vi "Configure List State.vi"(8 "error in":errorcluster, 10 "State":u16(ring) items=["OFF", " LIST1", " LIST2", " LIST3", " LIST4", " LIST5"], 11 "VISA resource name":refnum<visa-resource-name>) -> (0 "error out":errorcluster, 3 "VISA resource name out":refnum<visa-resource-name>)   [LabVIEW 2015, in "IT-M7700.lvlib"]
doc: "This command is used to set the mode of the List.\n<b>State</b>\n1~5 means to open the List function and call list1-list5, and OFF means to close the List function."
uses:
  <instrlib>/IT-M7700/IT-M7700.lvlib
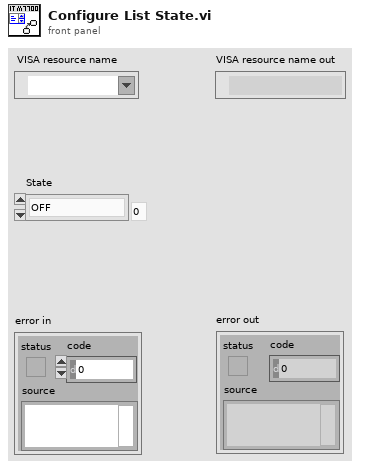
[diagram p1: front panel]
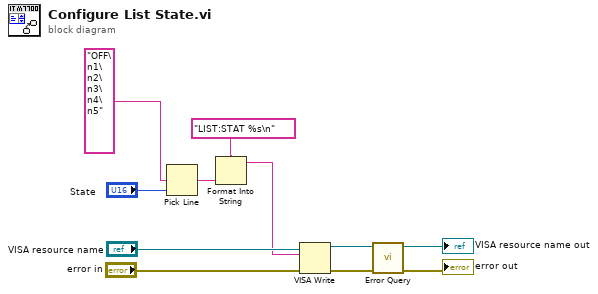
[diagram p0: block diagram]
diagram:
  n1 = Pick Line(multi-line string="OFF\n1\n2\n3\n4\n5", line index="State") -> (output string=w2:string)  [unwired: 1 in]
  n2 = Format Into String(format string="LIST:STAT %s\n", w2) -> (resulting string=w9:string)  [unwired: 2 in, 1 out]
  n3 = VISA Write(VISA resource name="VISA resource name", write buffer=w9, error in (no error)="error in") -> (VISA resource name out=w8:refnum<visa-resource-name>, error out=w7:errorcluster)  [unwired: 1 out]
  n4 = call <instrlib>:"Error Query.vi"("error in"=w7, "VISA resource name"=w8) -> ("error out"=→"error out":errorcluster, "VISA resource name out"=→"VISA resource name out":refnum<visa-resource-name>)  [unwired: 6 in, 2 out]
